vi "FTW-XML-Element-GetValue.vi"(0 "XML Node":refnum<k20>, 11 "error in":errorcluster) -> (4 "XML Node out":refnum<k20>, 6 "Node Text Value":string, 15 "error out":errorcluster)   [LabVIEW 2015]
uses:
  <resource>/objmgr/DOMUserDefRef.rc
panel:
  # "Inputs"
  # "Outputs"
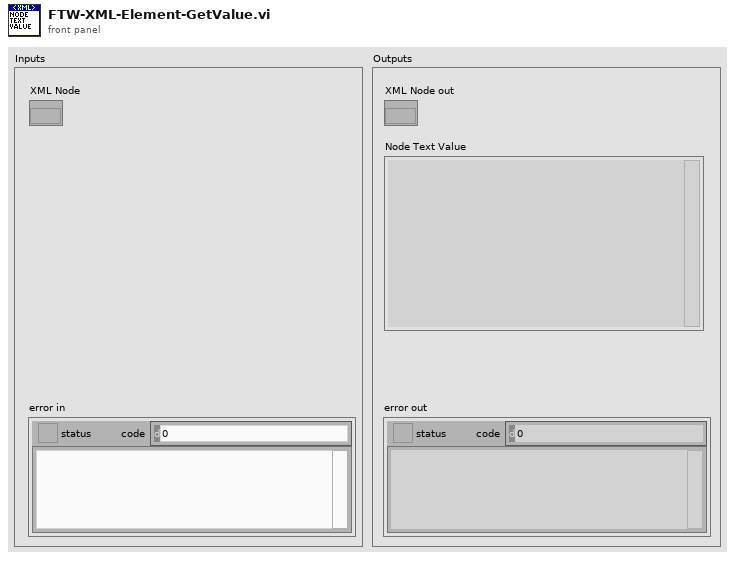
[diagram p1: front panel]
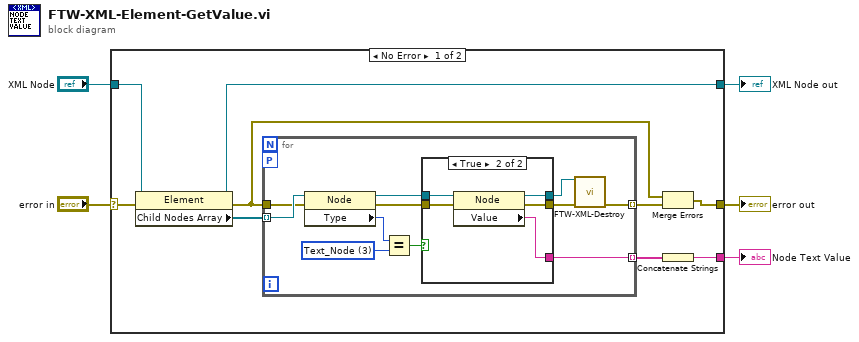
[diagram p0: block diagram]
diagram:
  n1 = case shown="No Error" "error in" {
    selector: "error in" -> [w14 w34]
    tunnel: [w10 w34] -> w5
    tunnel: "XML Node" -> [w13 w33]
    tunnel: [w12 w33] -> w2
    tunnel: [w11 _] -> w1
    frame No Error {
      n2 = property class="Element"(reference=w13, error in=w14) -> (reference out=w12:refnum<k20>, error out=w7:errorcluster, "Child Nodes Array"=w9:refnum<k20>[])
      n3 = for {
        tunnel: w9 -> [w25] mode=indexing
        tunnel: [w21] -> w8 mode=indexing
        workers-P: _ -> [_]
        tunnel: w7 -> [w24]
        tunnel: [w18] -> w6 mode=indexing
        w16 = 3 items=["Element_Node"=1, "Attribute_Node"=2, "Text_Node"=3, "CDATASection_Node"=4, "EntityReference_Node"=5, "Entity_Node"=6, "ProcessingInstruction_Node"=7, "Comment_Node"=8, "Document_Node"=9, "DocumentType_Node"=10, "DocumentFragment_Node"=11, "Notation_Node"=12] ("Node Type")
        n4 = property class="Node"(reference=w25, error in=w24) -> (reference out=w23:refnum<k20>, error out=w22:errorcluster, "Type"=w17:i32)
        n5 = Equal?(x=w17, y=w16) -> (x = y?=w15:bool)
        n6 = case shown="True" w15 {
          tunnel: w23 -> [w27 w32]
          tunnel: w22 -> [w26 w31]
          tunnel: [_ w30] -> w21
          tunnel: [w27 w29] -> w20
          tunnel: [w26 w28] -> w19
          frame False {
          }
          frame True {
            n7 = property class="Node"(reference=w32, error in=w31) -> (reference out=w29:refnum<k20>, error out=w28:errorcluster, "Value"=w30:string)
          }
        }
        n8 = call "FTW-XML-Destroy.vi"("XML Node"=w20, "error in"=w19) -> ("error out"=w18:errorcluster)  [unwired: 13 in]
      }
      n9 = Merge Errors(w7, w6) -> (w10:errorcluster)
      n10 = Concatenate Strings(w8) -> (w11:string)
    }
    frame Error {
    }
  }
  "error out" <- w5
  "XML Node out" <- w2
  "Node Text Value" <- w1
